vi "Main FPGA.vi"() -> ()   [LabVIEW 2015]
uses:
  <vilib>/Platform/TimedLoop/XDataNode/timing_clust.ctl
  <vilib>/Platform/TimedLoop/XDataNode/nitl_modes.ctl
  <vilib>/Platform/TimedLoop/XDataNode/wakeup.ctl
  <vilib>/rvi/Emulation/niFpgaGetClockAttributes.vi
  <vilib>/rvi/Emulation/niFpgaSctlEmulationGetInTimedLoop.vi
  <vilib>/rvi/Emulation/niFpgaEmulationReportErrorSimple.vi
  <vilib>/rvi/eio/common/nirviEmuTemplateMethod_errors.vi
  <vilib>/rvi/Emulation/niFpgaCriticalErrorInLSC.vi
  <vilib>/rvi/Emulation/niFpgaProcessEmulError.vi
  <vilib>/rvi/Emulation/niFpgaEmulationIsFPGAContextNoSignature.vi
  <vilib>/rvi/errors/niFpgaSetErrorForExecOnDevCompSimple.vi
  <vilib>/rvi/eio/common/nirviEmuReportErrorAndStop.vi
  <vilib>/rvi/DataTransferAndStorage/Container/Common/niFpgaContainerGetUniqueNameForEmu.vi
  <vilib>/rvi/FIFO/Fifo_Resource/nirvififoEmulationSetSize.vi
  <vilib>/rvi/FIFO/Fifo_Resource/nirviFifoEmulationQueueMgr.vi
  <instcachedir>/0/nirviFifoEmulationQueueMgr_E5CAEC123FF24DC58D834DCA3CDAA9B5.lvgen/nirviFifoEmulationQueueMgr_E5CAEC123FF24DC58D834DCA3CDAA9B5_001.vi
  <vilib>/rvi/FIFO/Fifo_Resource/nirvififoEmulationDetermineInputValidOut.vi
  <vilib>/rvi/FIFO/Fifo_Resource/nirvififoEmulationCreateLock.vi
  <vilib>/rvi/FIFO/Fifo_Resource/nirvififoEmulationObtainLock.vi
  <vilib>/rvi/FIFO/Fifo_Resource/nirvififoEmulationReleaseLock.vi
  <vilib>/rvi/occurrence/nirviWaitOnOccurrenceBase.vi
  <vilib>/rvi/errors/nirviReportUnexpectedCaseInternalError.vi
  <vilib>/rvi/errors/nirviReportUnexpectedCaseInternalError (U32).vi
  <vilib>/Utility/error.llb/Clear Errors.vi
  <vilib>/eio/EIONode/EIONode.xnode
  <vilib>/rvi/DataTransferAndStorage/Container/XNode/niFpgaContainer.xnode
  <vilib>/rvi/FIFO/Fifo_Resource/nirvififoEmulationWrite.vi
  <vilib>/rvi/FIFO/Fifo_Resource/nirvififoEmulationRead.vi
  <vilib>/Platform/TimedLoop/XDataNode/XDataNode.xnode
  <vilib>/Platform/TimedLoop/XDataNode/XDNodeRunTimeDep.lvlib
panel:
  in  "stop bits (10: 1 bit)":u16(ring)=10 items=["1.0"=10, "1.5"=15, "2.0"=20]
  in  "parity (0:none)":enum16{"None", "Odd", "Even", "Mark", "Space"}(ring)
  in  "data bits (8)":i32=8 min=5 max=8 step=1
  out "Read: Char":u8
  out "Read: New Data":bool
  in  "stop":bool
  in  "Invert Polarity?":bool
  in  "baud rate (9600)":u32=9600
  in  "Write: Char":u8
  in  "Write: Data Written":bool
  out "Reset stop 25":bool
  in  "DIO22":bool
  in  "DIO21":bool
  in  "YAW 3":fxp<+,32,0>=0.5 caption="duty cycle (periods)"
  in  "YAW 2":fxp<+,32,0>=0.5 caption="duty cycle (periods)"
  in  "ROLL 3":fxp<+,32,0>=0.5 caption="duty cycle (periods)"
  in  "ROLL 2":fxp<+,32,0>=0.5 caption="duty cycle (periods)"
  in  "PITCH 3":fxp<+,32,0>=0.5 caption="duty cycle (periods)"
  in  "PITCH 2":fxp<+,32,0>=0.5 caption="duty cycle (periods)"
  in  "YAW1":fxp<+,32,0>=0.5 caption="duty cycle (periods)"
  in  "ROLL1":fxp<+,32,0>=0.5 caption="duty cycle (periods)"
  in  "PITCH 1":fxp<+,32,0>=0.5 caption="duty cycle (periods)"
  in  "frequency (periods/tick)":fxp<+,32,0>=1.0338844731450081e-05
  in  "SAFETY ON":bool
  out "STOP ??":bool
  out "System Reset":bool
  out "Czas od ostatniego sygnalu":u64
  in  "watchdog":bool
  in  "dozwolony czas pomiedzy watchdogiem":u64=5000
  in  "wlacz watchdoga":bool
  in  "RESET STM":bool
  out "temperatura":sgl
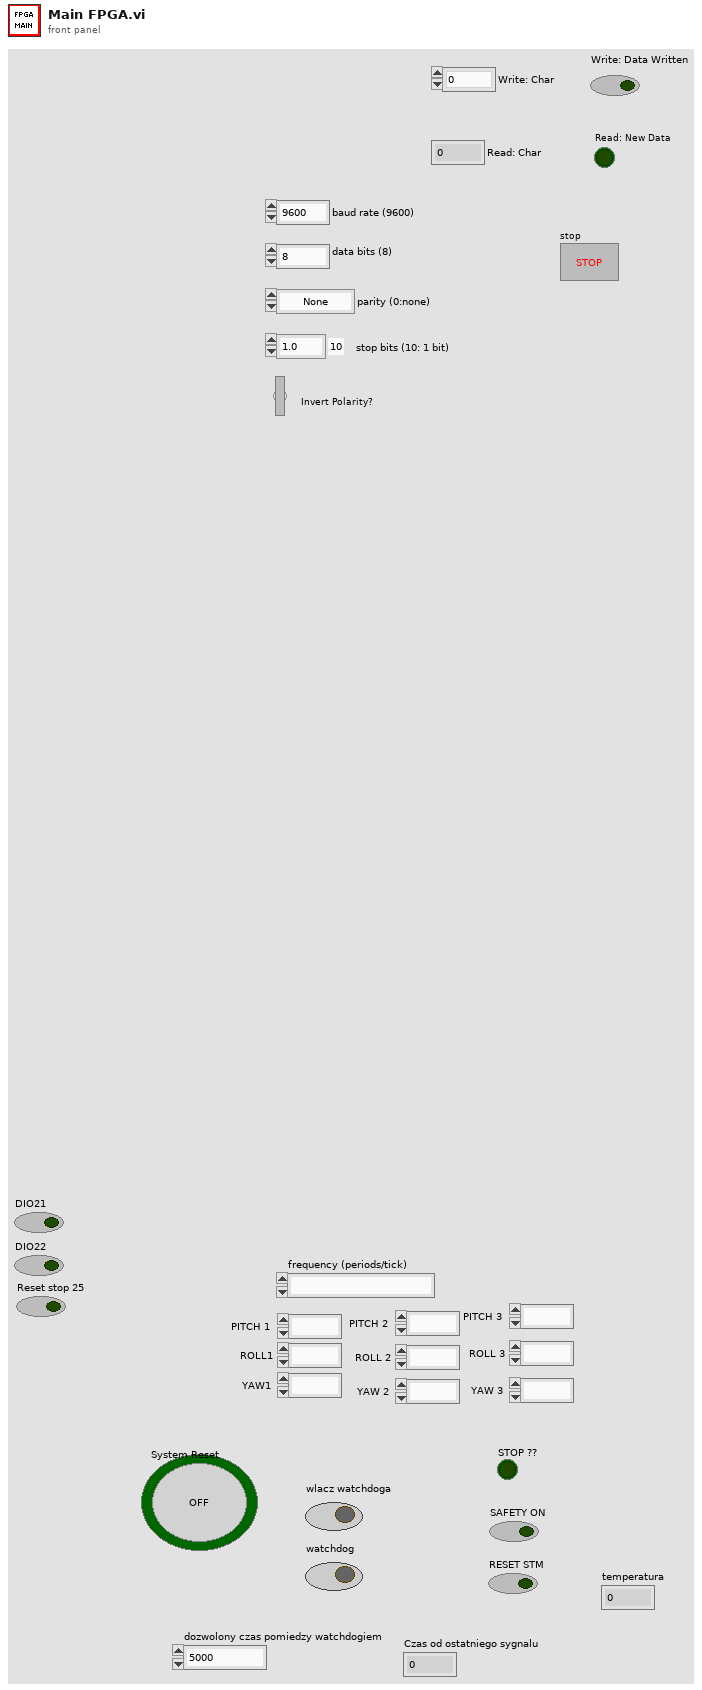
[diagram p1: front panel]
types:
  T1 = typedef "XDNodeRunTimeDep.lvlib/timing_clust.ctl" = cluster{"Expected End [f-1]":u64, "Actual End [f-1]":u64, "Finished Late? [f-1]":bool, "Expected End [i-1]":u64, "Actual End [i-1]":u64, "Finished Late? [i-1]":bool, "Expected Start [i]":u64, "Actual Start [i]":u64, "Expected Start [f]":u64, "Actual Start [f]":u64, "Source Name":string, "Structure Name":string, "Period":i64, "Deadline":i64, "Offset":i64, "Start":i64, "Priority":i32, "Timeout":i32, "Mode":T2, "Wakeup Reason":T3, "Error":errorcluster, "Source Type":string, "Secondary Source Type":string, "Global End Time":u64, "Global Start Time":u64, "Frame Duration":u64, "Iteration Duration":u64, "Assigned CPU":i32, "I/O Scan Engine Mode":u32}
  T2 = typedef "XDNodeRunTimeDep.lvlib/nitl_modes.ctl" = enum32{"No Change", "Process missed periods, maintain original phase", "Discard missed periods, maintain original phase", "Process missed periods, ignore original phase", "Discard missed periods, ignore original phase"}
  T3 = typedef "XDNodeRunTimeDep.lvlib/wakeup.ctl" = enum32{"Normal", "Aborted", "Asynchronous wakeup", "Timing source error", "Timed loop error", "Timeout"}
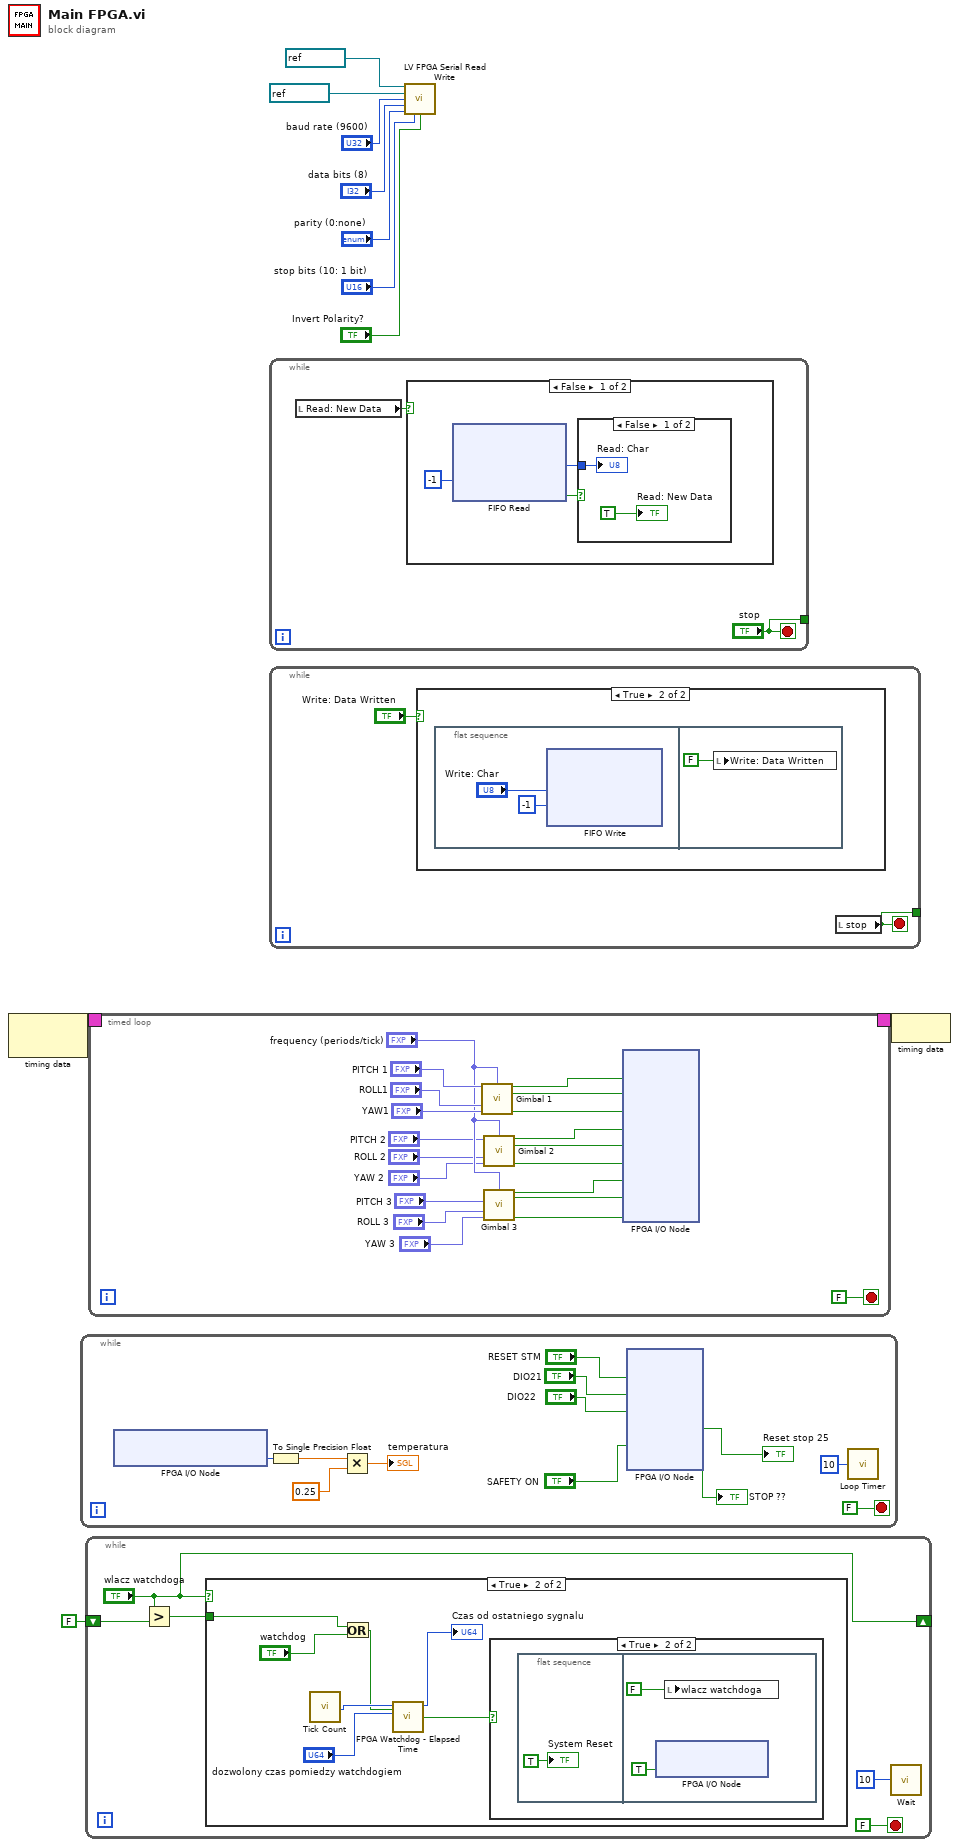
[diagram p0: block diagram]
diagram:
  n1 = node-c288() -> (w9:T1)  [unwired: 1 in]
  n2 = while {
    stop <- FALSE stop-if-true
    n3 = xnode "FPGA I/O Node"() -> ("Chassis Temperature"=w18:i16)  [unwired: 1 in, 1 out]
    n4 = To Single Precision Float(number=w18) -> (single precision float=w20:sgl)
    n5 = Multiply(x=w20, y=sgl 0.25) -> (x*y=→"temperatura":sgl)
    n6 = xnode "FPGA I/O Node"("DIO20"="RESET STM", "DIO21"="DIO21", "DIO22"="DIO22", "DIO26"="SAFETY ON") -> ("DIO25"=→"Reset stop 25":bool, "DIO27"=→"STOP ??":bool)  [unwired: 6 in, 6 out]
    n7 = call "Loop Timer"("Count(uSec)"=u32 10) -> ()  [unwired: 1 out]
  }
  n8 = while {
    shift-right: ["wlacz watchdoga"] -> _
    shift-left: FALSE -> [w24]
    stop <- FALSE stop-if-true
    n9 = Greater?(x="wlacz watchdoga", y=w24) -> (0:w25:bool)
    n10 = case shown="True" "wlacz watchdoga" {
      tunnel: w25 -> [_ w34]
      frame False {
      }
      frame True {
        n11 = call "Tick Count"() -> ("Tick Count(mSec)"=w31:u32)
        n12 = Or(x=w34, y="watchdog") -> (x .or. y?=w30:bool)
        n13 = call "FPGA Watchdog - Elapsed Time.vi"("Reset"=w30, "Timeout Period"="dozwolony czas pomiedzy watchdogiem", "Current Time"=w31) -> ("Timeout"=w28:bool, "Elapsed Time"=→"Czas od ostatniego sygnalu":u64)  [unwired: 7 in]
        n14 = case shown="True" w28 {
          frame False {
          }
          frame True {
            n15 = flat-sequence {
              frame #0 {
                "System Reset" <- TRUE ("System Reset")
              }
              frame #1 {
                n16 = xnode "FPGA I/O Node"("System Reset"=TRUE) -> ()  [unwired: 1 in, 1 out]
                n17 = local write "wlacz watchdoga"(FALSE ("System Reset")) -> ()
              }
            }
          }
        }
      }
    }
    n18 = call "Wait"("Count(uSec)"=u32 10) -> ()  [unwired: 1 out]
  }
  n19 = timed-loop {
    timing: w9 -> [_]
    timing-out: [_] -> w8
    stop <- FALSE stop-if-true
    n20 = call "Gimbal 1.vi"("PITCH 1"="PITCH 1", "frequency (periods/tick)"="frequency (periods/tick)", "ROLL1"="ROLL1", "YAW1"="YAW1") -> ("DIO 7"=w56:bool, "DIO 8"=w55:bool, "DIO 9"=w54:bool)  [unwired: 9 in]
    n21 = call "Gimbal 2.vi"("frequency (periods/tick)"="frequency (periods/tick)", "PITCH 2"="PITCH 2", "ROLL2"="ROLL 2", "YAW 2"="YAW 2") -> ("DIO 10"=w50:bool, "DIO 11"=w49:bool, "DIO 12"=w48:bool)  [unwired: 9 in]
    n22 = call "Gimbal 3.vi"("frequency (periods/tick)"="frequency (periods/tick)", "PITCH 3"="PITCH 3", "ROLL 3"="ROLL 3", "YAW 3"="YAW 3") -> ("DIO 13"=w47:bool, "DIO 14"=w46:bool, "DIO 15"=w45:bool)  [unwired: 9 in]
    n23 = xnode "FPGA I/O Node"("DIO7"=w56, "DIO8"=w55, "DIO9"=w54, "DIO10"=w50, "DIO11"=w49, "DIO12"=w48, "DIO13"=w47, "DIO14"=w46, "DIO15"=w45) -> ()  [unwired: 9 in, 9 out]
  }
  n24 = while {
    tunnel: ["stop"] -> _
    stop <- "stop" stop-if-true
    n25 = local read "Read: New Data"() -> (w61:bool)
    n26 = case shown="False" w61 {
      frame False {
        n27 = xnode ("FIFO Read")("Timeout"=-1) -> ("Element"=w62:u8, "Timed Out?"=w63:bool)  [unwired: 1 in, 1 out]
        n28 = case shown="False" w63 {
          tunnel: w62 -> [w66 _]
          frame False {
            "Read: Char" <- w66
            "Read: New Data" <- TRUE ("Read: New Data")
          }
          frame True {
          }
        }
      }
      frame True {
      }
    }
  }
  n29 = while {
    tunnel: [w67] -> _
    stop <- w67 stop-if-true
    n30 = case shown="True" "Write: Data Written" {
      frame False {
      }
      frame True {
        n31 = flat-sequence {
          frame #0 {
            n32 = xnode ("FIFO Write")("Element"="Write: Char", "Timeout"=-1) -> ()  [unwired: 1 in, 2 out]
          }
          frame #1 {
            n33 = local write "Write: Data Written"(FALSE ("Write: Data Written")) -> ()
          }
        }
      }
    }
    n34 = local read "stop"() -> (w67:bool)
  }
  n35 = call "LV FPGA Serial Read Write.vi"("Transmit"=refnum<k21> "DIO24", "Receive"=refnum<k21> "DIO23", "baud rate (9600)"="baud rate (9600)", "data bits (8)"="data bits (8)", "parity (0:none)"="parity (0:none)", "stop bits (10: 1 bit)"="stop bits (10: 1 bit)", "Invert Polarity?"="Invert Polarity?") -> ()  [unwired: 9 out]
  n36 = node-c288(w8) -> ()
